vi "Draw.vi"(8 "error in (no error)":errorcluster, 11 "Line in":refnum<class "Line.lvclass">) -> (0 "error out":errorcluster, 2 "Picture":picture, 3 "Line out":refnum<class "Line.lvclass">)   [LabVIEW 2015, in "LV Image Editor Framework.lvlib" / "Line.lvclass"]
uses:
  Line.lvclass
  Shape/Shape.lvclass/Shape.ctl
  Line.lvclass/Line.ctl
  Shape/Shape.lvclass
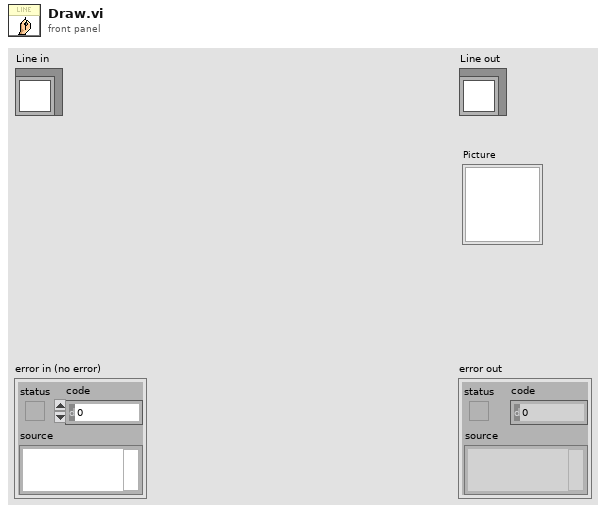
[diagram p1: front panel]
types:
  T1 = cluster{"Left":i32, "Top":i32, "Right":i32, "Bottom":i32}
  T2 = cluster{"Width":u16, "Style":enum32{"Solid", "Dash", "Dot", "DashDot", "DashDotDot"}}
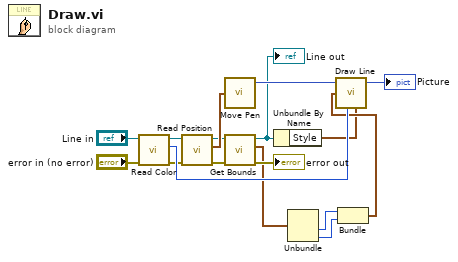
[diagram p0: block diagram]
diagram:
  n1 = call "Read Color.vi"("error in (no error)"="error in (no error)", "Shape in"="Line in") -> ("error out"=w12:errorcluster, "Color"=w14:u32, "Shape out"=w15:refnum<class "Line.lvclass">)  [unwired: 7 in]
  n2 = call-dynamic "Read Position.vi"("error in (no error)"=w12, "Shape in"=w15) -> ("error out"=w11:errorcluster, "Position"=w16:cluster{"Left":i32, "Top":i32}, "Shape out"=w4:refnum<class "Line.lvclass">)  [unwired: 7 in]
  n3 = call <vilib>:"Move Pen.vi"("new position"=w16) -> ("new picture"=w17:picture)  [unwired: 4 in]
  n4 = call "Get Bounds.vi"("error in (no error)"=w11, "Shape in"=w4) -> ("error out"=→"error out":errorcluster, "Bounds"=w8:T1, "Shape out"=w1:refnum<class "Line.lvclass">)  [unwired: 7 in]
  "Line out" <- w1
  n5 = Unbundle By Name(w1) -> ("Style"=w2:T2)
  n6 = Unbundle(w8) -> ("Right"=w7:i32, "Bottom"=w6:i32)  [unwired: 2 out]
  n7 = Bundle("Right"=w7, "Bottom"=w6) -> (w5:cluster{"Right":i32, "Bottom":i32})  [unwired: 1 in]
  n8 = call <vilib>:"Draw Line.vi"("picture"=w17, "end point"=w5, "color(black)"=w14, "pen"=w2) -> ("new picture"=→"Picture":picture)  [unwired: 5 in]
